vi "GetReferenceByUID.vi"(3 "error in (no error)":errorcluster, 4 "objectClass":string="GObject", 5 "UID":i32, 6 "targetVI":refnum<vi>) -> (0 "error out":errorcluster, 1 "refNum":refnum<vi>, 2 "dup targetVI":refnum<vi>)   [LabVIEW 2013]
uses:
  <vilib>/Utility/traverseref.llb/TRef TravTarget.ctl
panel:
  out "all":cluster{"UID":i32, "objref":refnum<vi>}[](array[cluster])
  out "cache":T1(array[cluster])
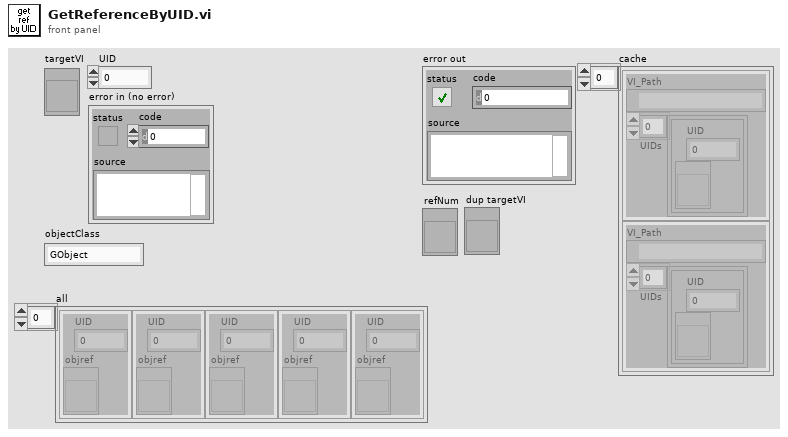
[diagram p1: front panel]
types:
  T1 = cluster{"VI_Path":path, "UIDs":cluster{"UID":i32, refnum<vi>}[]}[]
  T2 = typedef "TRef TravTarget.ctl" = enum16{"FP", "BD", "Other"}
  T3 = cluster{"Path":path, cluster{"UID":i32, "objref":refnum<vi>}[]}
  T4 = cluster{"Path":path, cluster{"UID":i32, "objref":refnum<vi>}[]}[]
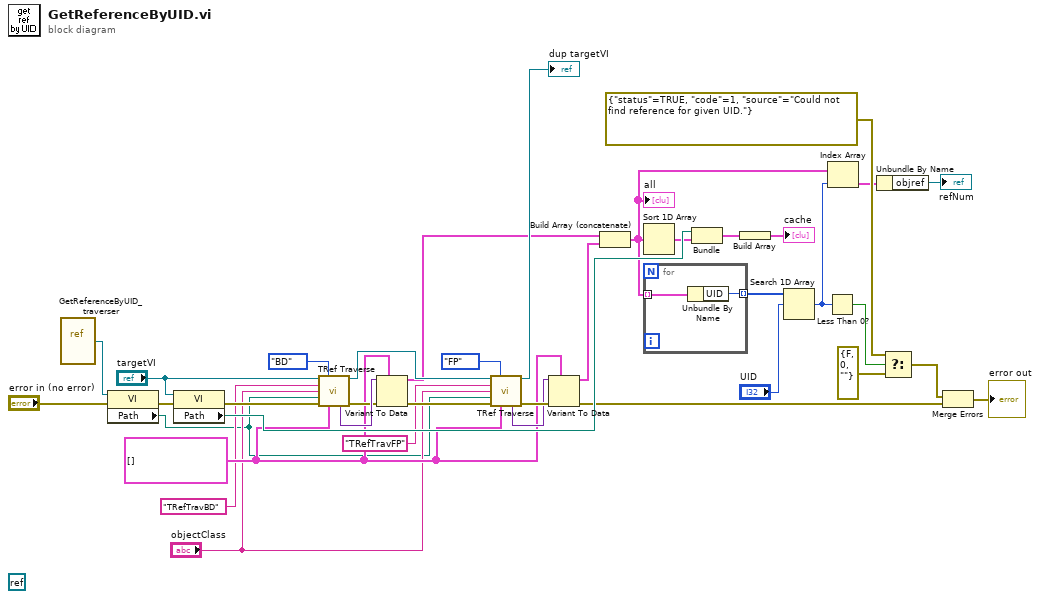
[diagram p0: block diagram]
diagram:
  w7 = cluster{"UID":i32, "objref":refnum<vi>}[] [] ("appended array")
  (unwired) refnum<k0> refnum
  n1 = vi-ref "GetReferenceByUID_traverser.vi"() -> (w29:refnum<vi>)
  n2 = property class="VI"(reference=w29, error in="error in (no error)") -> (error out=w20:errorcluster, "Path"=w3:path)  [unwired: 1 out]
  n3 = property class="VI"(reference="targetVI", error in=w20) -> (error out=w19:errorcluster, "Path"=w33:path)  [unwired: 1 out]
  n4 = call <vilib>:"TRef Traverse.vi"("VI Refnum"="targetVI", "Traverse Target"=TRef_TravTarget."BD", "OpName (\"TRefTrav\")"="TRefTravBD" ("OpName (\"TRefTrav\")"), "Class Name"="objectClass", "Callback Path"=w3, "error in (no error)"=w19, "ContextData type"=w7) -> ("dup VI Refnum"=w14:refnum<vi>, "ContextData"=w28:variant, "error out"=w15:errorcluster)  [unwired: 6 in]
  n5 = Variant To Data(error in=w15, type=w7, Variant=w28) -> (data=w9:cluster{"UID":i32, "objref":refnum<vi>}[], error out=w13:errorcluster)
  n6 = call <vilib>:"TRef Traverse.vi"("VI Refnum"=w14, "Traverse Target"=TRef_TravTarget."FP", "OpName (\"TRefTrav\")"="TRefTravFP" ("OpName (\"TRefTrav\")"), "Class Name"="objectClass", "Callback Path"=w3, "error in (no error)"=w13, "ContextData type"=w7) -> ("dup VI Refnum"=→"dup targetVI":refnum<vi>, "ContextData"=w8:variant, "error out"=w12:errorcluster)  [unwired: 6 in]
  n7 = Variant To Data(error in=w12, type=w7, Variant=w8) -> (data=w6:cluster{"UID":i32, "objref":refnum<vi>}[], error out=w10:errorcluster)
  n8 = Build Array (concatenate)(w9, w6) -> (w1:cluster{"UID":i32, "objref":refnum<vi>}[])
  "all" <- w1
  n9 = Sort 1D Array(array=w1) -> (sorted array=w32:cluster{"UID":i32, "objref":refnum<vi>}[])
  n10 = for {
    tunnel: [w39] -> w25 mode=indexing
    tunnel: w1 -> [w38] mode=indexing
    n11 = Unbundle By Name(w38) -> ("UID"=w39:i32)
  }
  n12 = Bundle("Path"=w33, w32) -> (w31:T3)  [unwired: 1 in]
  n13 = Build Array(w31) -> (→"cache":T4)
  n14 = Search 1D Array(1D array=w25, element="UID") -> (index of element=w18:i32)  [unwired: 1 in]
  n15 = Less Than 0?(x=w18) -> (x < 0?=w17:bool)
  n16 = Index Array(array=w1, index=w18) -> (element=w23:cluster{"UID":i32, "objref":refnum<vi>})
  n17 = Unbundle By Name(w23) -> ("objref"=→"refNum":refnum<vi>)
  n18 = Select(t=errorcluster {"status"=TRUE, "code"=1, "source"="Could not find reference for given UID."}, s=w17, f=errorcluster {"status"=FALSE, "code"=0, "source"=""}) -> (s? t:f=w36:errorcluster)
  n19 = Merge Errors(w36, w10) -> (→"error out":errorcluster)
